vi "TapeWaitForTapeMonitorCam.vi"(8 "error in (no error)":errorcluster, 11 "TapeDrive in":refnum<class "TapeDrive.lvclass">) -> (0 "error out":errorcluster, 1 "maxCounts":dbl[](graph), 2 "MaxCountsOk":bool, 3 "TapeDrive out":refnum<class "TapeDrive.lvclass">)   [LabVIEW 2020, in "TapeDrive.lvclass"]
uses:
  TapeDrive.lvclass
  TapeDrive.lvclass/TapeDrive.ctl
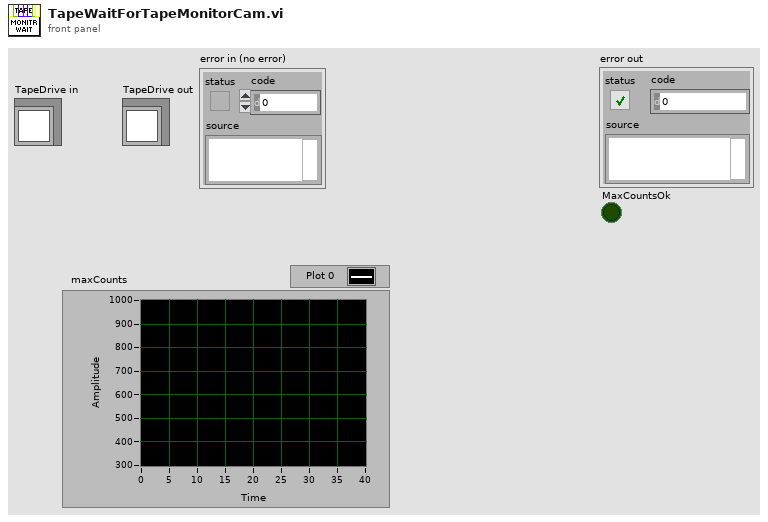
[diagram p1: front panel]
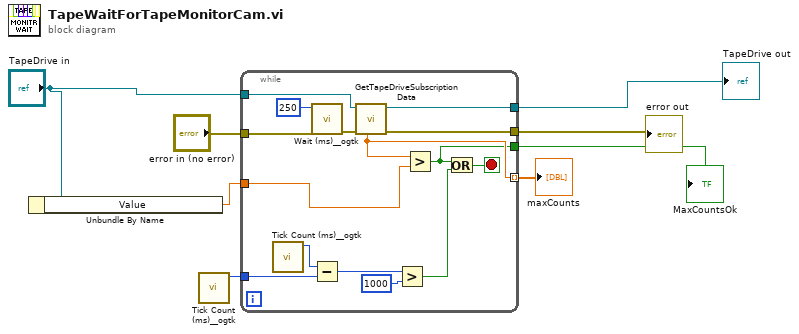
[diagram p0: block diagram]
diagram:
  n1 = Unbundle By Name("TapeDrive in") -> ("Value"=w2:dbl)
  n2 = call "Tick Count (ms)__ogtk.vi"() -> ("millisecond timer value"=w6:u32)  [unwired: 10 in, 1 out]
  n3 = while {
    tunnel: "TapeDrive in" -> [w23]
    tunnel: [w22] -> w7
    tunnel: [w18] -> w8 mode=indexing
    tunnel: [w19] -> w4
    tunnel: w6 -> [w16]
    tunnel: "error in (no error)" -> [w11]
    tunnel: w2 -> [w10]
    tunnel: [w9] -> w1
    stop <- w12 stop-if-true
    n4 = call "Tick Count (ms)__ogtk.vi"() -> ("millisecond timer value"=w17:u32)  [unwired: 10 in, 1 out]
    n5 = call "Wait (ms)__ogtk.vi"("error in (no error)"=w11, "milliseconds to wait"=u32 250) -> ("error out"=w21:errorcluster)  [unwired: 8 in, 1 out]
    n6 = Subtract(x=w17, y=w16) -> (x-y=w15:u32)
    n7 = call "GetTapeDriveSubscriptionData.vi"("error in (no error)"=w21, "TapeDrive in"=w23) -> ("error out"=w19:errorcluster, "TapeDrive in 2"=w22:refnum<class "TapeDrive.lvclass">, "TapeMonMaxCounts"=w18:dbl)  [unwired: 3 in, 4 out]
    n8 = Greater?(x=w15, y=u32 1000) -> (0:w13:bool)
    n9 = Greater?(x=w18, y=w10) -> (0:w9:bool)
    n10 = Or(x=w9, y=w13) -> (x .or. y?=w12:bool)
  }
  "maxCounts" <- w8
  "TapeDrive out" <- w7
  "error out" <- w4
  "MaxCountsOk" <- w1
